vi "FW Get Position.vi"(0 "Notifier Name In":string, 11 "Error In":errorcluster) -> (4 "Notifier Name Out":string, 8 "Position":i32, 15 "Error Out":errorcluster)   [LabVIEW 2020]
uses:
  FW Type Defs/FW Notifier Type.ctl
  FW Type Defs/FW Actions.ctl
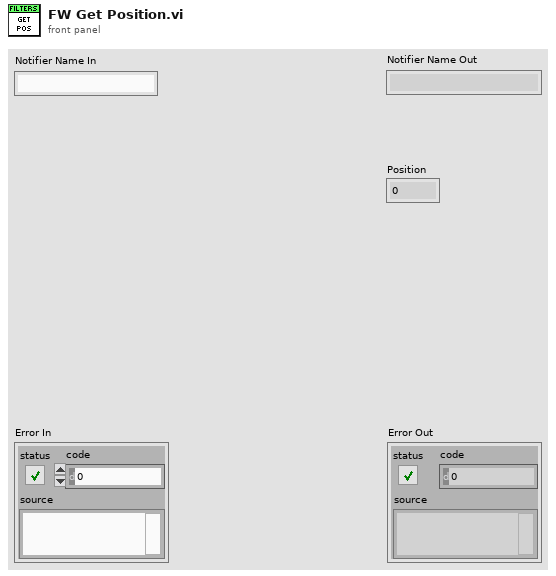
[diagram p1: front panel]
types:
  T1 = typedef "FW Notifier Type.ctl" = cluster{"Actions":T2, "Set Position":u8, "Actual Position":u8, "Speed":dbl, "Num Positions":u8, "Received":bool}
  T2 = typedef "FW Actions.ctl" = enum16{"Set Position", "Get Position", "Get Num Positions", "Set Speed", "Confirm Pos", "Quit"}
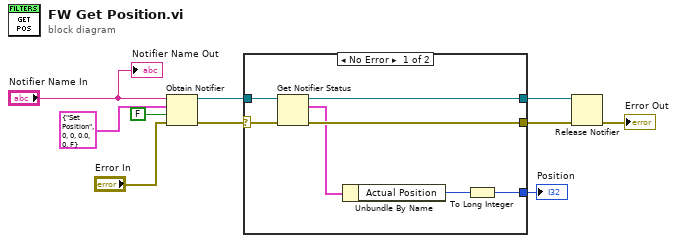
[diagram p0: block diagram]
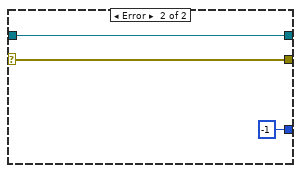
[diagram p2: hidden frame]
diagram:
  n1 = Obtain Notifier(name (unnamed)="Notifier Name In", notification data type=T1 {"Actions"=enum."Set Position", "Set Position"=0, "Actual Position"=0, "Speed"=0.0, "Num Positions"=0, "Received"=FALSE} ("FW102C Note Type"), create if not found? (T)=FALSE, error in (no error)="Error In") -> (notifier out=w7:refnum<notifier>, error out=w8:errorcluster)  [unwired: 1 out]
  n2 = case shown="No Error" w8 {
    selector: w8 -> [w16 w20]
    tunnel: w7 -> [w17 w19]
    tunnel: [w14 w20] -> w4
    tunnel: [w15 w19] -> w5
    tunnel: [w11 -1] -> w1
    frame No Error {
      n3 = Get Notifier Status(notifier=w17, error in (no error)=w16) -> (notifier out=w15:refnum<notifier>, current notification=w13:T1, error out=w14:errorcluster)  [unwired: 2 out]
      n4 = Unbundle By Name(w13) -> ("Actual Position"=w12:u8)
      n5 = To Long Integer(number=w12) -> (32bit integer=w11:i32)
    }
    frame Error {
    }
  }
  "Position" <- w1
  n6 = Release Notifier(notifier=w5, error in (no error)=w4) -> (error out=→"Error Out":errorcluster)  [unwired: 1 in, 2 out]
  "Notifier Name Out" <- "Notifier Name In"
